vi "OperateOnAnalogOutput.vi"(2 "error in (no error)":errorcluster, 3 "operation":enum16{"start", "state", "abort"}(ring)) -> (0 "error out":errorcluster, 1 "generation complete":bool)   [LabVIEW 2009]
uses:
  StageType.ctt
  AO Write (waveform).vi
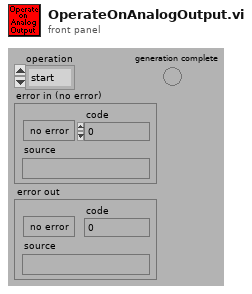
[diagram p1: front panel]
types:
  T1 = enum16{"Get Type", "Set Type", "GetStageInit", "GetWriteStageSetting", "GetInitializeStageOutput", "GetSetAxisPosition", "GetSetPos", "GetSetupStage", "HaltStageOutput", "InitializeStageOutputChannels"}
  T2 = typedef "StageType.ctt" = enum16{"PI analogue", "PI 712 TCP/IP", "Märzhäuser", "PI analogue step", "PI 712 USB"}
  T3 = enum16{"Get Type", "Set Type", "GetStageInit", "GetWriteStageSetting", "GetInitializeStageOutput", "GetSetAxisPosition", "GetSetPos", "GetSetupStage", "HaltStageOutput"}
  T4 = typedef "AnalogSettings.ctt" = cluster{"PCI 671x Device Number":u32, "Samples per Unit":u32}
  T5 = typedef "TimingInfo.ctt" = cluster{"Fs":dbl, "#s":dbl}
  T6 = typedef "AnalogOutput.ctt" = waveform(dbl)[]
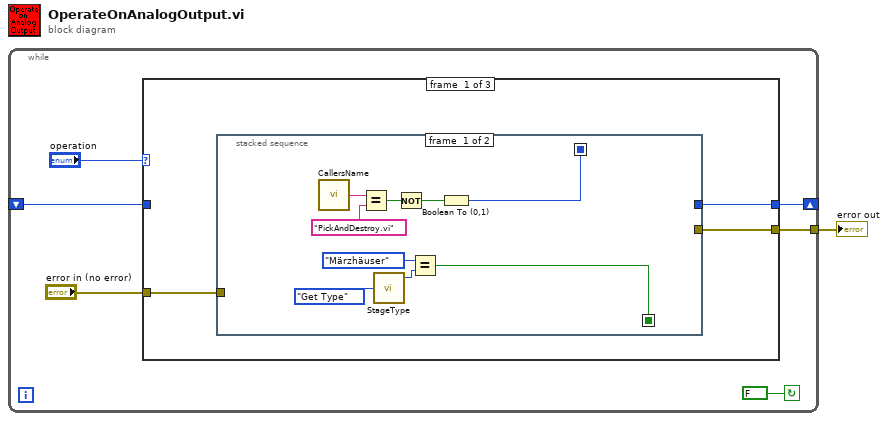
[diagram p0: block diagram]
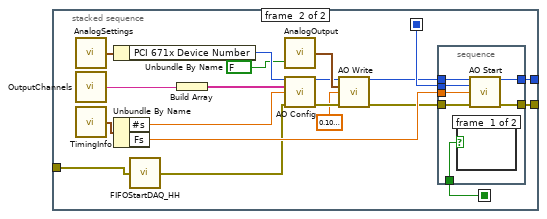
[diagram p2: hidden frame]
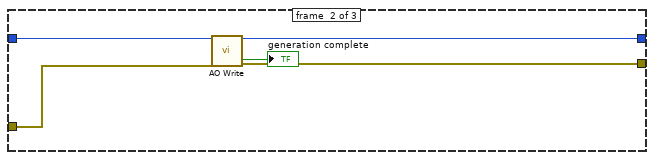
[diagram p4: hidden frame]
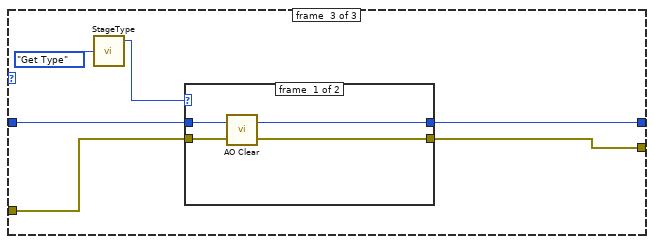
[diagram p5: hidden frame]
diagram:
  n1 = while {
    shift-right: [w5] -> _
    shift-left: _ -> [w4]
    tunnel: [w2] -> w1
    stop <- FALSE continue-if-true
    n2 = case shown="\"abort\"" "operation" {
      tunnel: [w10 w50 w56] -> w5
      tunnel: w4 -> [_ w51 w57]
      tunnel: "error in (no error)" -> [w8 w48 w55]
      tunnel: [w9 w47 w54] -> w2
      frame #0 {
        n3 = stacked-sequence {
          seq-local: [w16 _] -> [_ w27]
          seq-local: [w11 _] -> [_ w24]
          tunnel: [_ w31] -> w10
          tunnel: [_ w30] -> w9
          tunnel: w8 -> [_ w21]
          frame #0 {
            n4 = call "CallersName.vi"() -> ("Callers Name out"=w19:string)  [unwired: 2 in]
            n5 = Equal?(x=w19, y="PickAndDestroy.vi") -> (x = y?=w17:bool)
            n6 = call "StageType.vi"("Function"=T1."Get Type") -> ("Stage Type (output)"=w12:T2)  [unwired: 2 in, 2 out]
            n7 = Not(x=w17) -> (.not. x?=w15:bool)
            n8 = Equal?(x=StageType.ctt."Märzhäuser" ("Stage Type (input)"), y=w12) -> (x = y?=w11:bool)
            n9 = Boolean To (0,1)(Boolean=w15) -> (0, 1=w16:i16)
          }
          frame #1 {
            n10 = call "AnalogSettings.vi"() -> ("Analog Settings (output)"=w38:T4)  [unwired: 2 in]
            n11 = call "OutputChannels.vi"() -> ("Output Channels (output)"=w23:tag)  [unwired: 2 in]
            n12 = call "TimingInfo.vi"() -> ("Timing Info (output)"=w35:T5)  [unwired: 2 in]
            n13 = Unbundle By Name(w38) -> ("PCI 671x Device Number"=w37:u32)
            n14 = Unbundle By Name(w35) -> ("#s"=w28:dbl, "Fs"=w29:dbl)
            n15 = call "FIFOStartDAQ_HH.vi"("error in (no error)"=w21) -> ("error out"=w20:errorcluster)
            n16 = Build Array(w23) -> (w36:tag[])
            n17 = call "AnalogOutput.vi"("Get/Set"=FALSE) -> ("Analog Output (output)"=w39:T6)  [unwired: 1 in]
            n18 = call <vilib>:"AO Config.vi"("device (1)"=w37, "channels (0)"=w36, "buffer size (1000 updates)"=w28, "error in (no error)"=w20) -> ("taskID"=w34:u32, "error out"=w33:errorcluster)  [unwired: 9 in, 1 out]
            n19 = call-poly "AO Write.vi"("taskID in"=w34, "waveform data"=w39, "time limit in sec (no change:-1)"=sgl 0.1, "error in (no error)"=w33) -> ("taskID out"=w26:u32, "error out"=w25:errorcluster)  [unwired: 7 in, 3 out]
            n20 = stacked-sequence {
              tunnel: [w46] -> w31
              tunnel: [w45] -> w30
              tunnel: w29 -> [w44]
              tunnel: w27 -> [w43]
              tunnel: w26 -> [w42]
              tunnel: w25 -> [w41]
              tunnel: w24 -> [w40]
              frame #0 {
                n21 = case shown="False" w40 {
                  frame #0 {
                  }
                  frame #1 {
                  }
                }
                n22 = call "AO Start.vi"("taskID in"=w42, "number of buffer iterations (1)"=w43, "update rate (1000 updates/sec)"=w44, "error in (no error)"=w41) -> ("taskID out"=w46:u32, "error out"=w45:errorcluster)  [unwired: 9 in, 1 out]
              }
            }
          }
        }
      }
      frame #1 {
        n23 = call-poly "AO Write.vi"("taskID in"=w51, "error in (no error)"=w48) -> ("taskID out"=w50:u32, "generation complete"=→"generation complete":bool, "error out"=w47:errorcluster)  [unwired: 9 in, 2 out]
      }
      frame #2 {
        n24 = call "StageType.vi"("Function"=T3."Get Type") -> ("Stage Type (output)"=w52:T2)  [unwired: 2 in, 2 out]
        n25 = case shown="\"PI 712 TCP/IP\", \"PI 712 USB\"" w52 {
          tunnel: w57 -> [w61 w63]
          tunnel: [w60 w63] -> w56
          tunnel: w55 -> [w59 w62]
          tunnel: [w58 w62] -> w54
          frame #0 {
            n26 = call "AO Clear.vi"("error in (no error)"=w59, "taskID in"=w61) -> ("error out"=w58:errorcluster, "taskID out"=w60:u32)  [unwired: 4 in]
          }
          frame #1 {
          }
        }
      }
    }
  }
  "error out" <- w1
